vi "Send Email.vi"(8 "error in":errorcluster, 9 "Email Configuration":T2={"Subject"="Checking the Toolkit", "Body"="Please reply!", "Recipients Email Addresses"="", "CC - Optional"=[""]}, 10 "Sender's Configuration":T1={"Outgoing Mail Server (SMTP)"="smtp.gmail.com", "Port"=587, "Sender's Email"="", "Email Password"="", "Sender's Name"=""}, 11 "Attachment(optional)":path) -> (0 "error out":errorcluster)   [LabVIEW 2016]
doc: "Send Email VI sends email to specified accounts(depending on the server and port mentioned) with an optional attachment. Note that the default settings are for Gmail."
uses:
  controls/Email Configuration.ctl
  controls/Receipants Email Address.ctl
  controls/Sender's Configuration.ctl
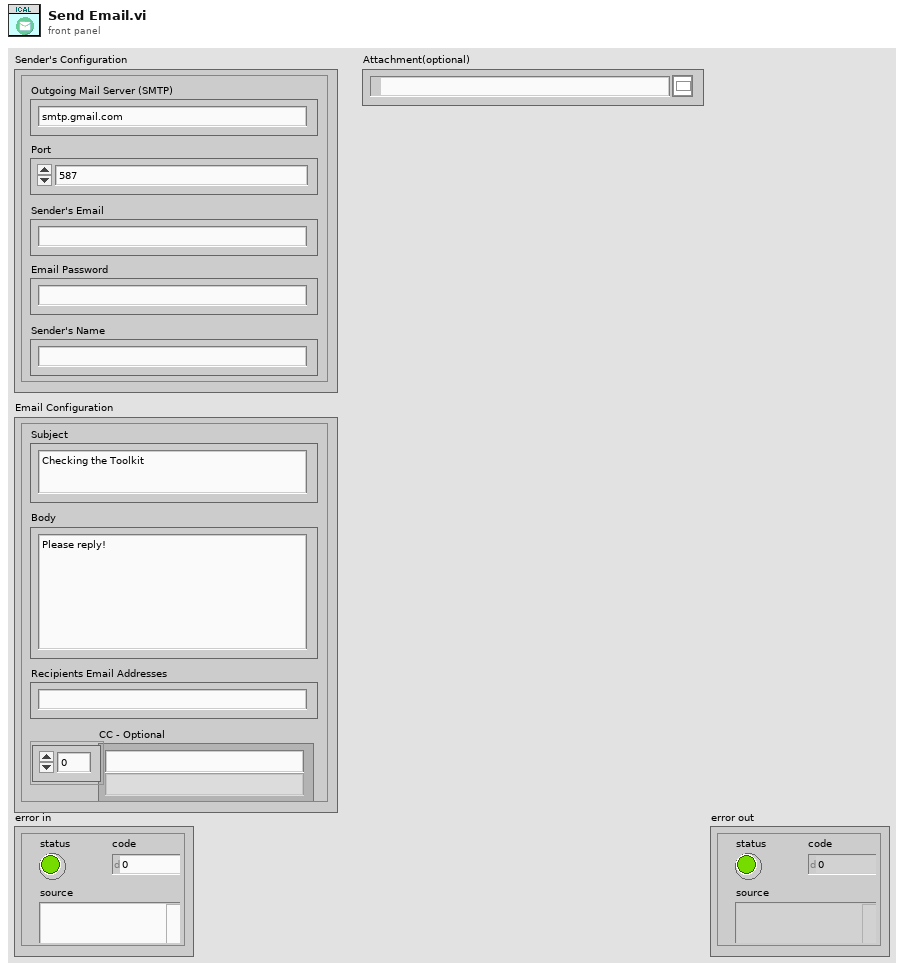
[diagram p1: front panel]
types:
  T1 = typedef "Sender's Configuration.ctl" = cluster{"Outgoing Mail Server (SMTP)":string, "Port":i32, "Sender's Email":string, "Email Password":string, "Sender's Name":string}
  T2 = typedef "Email Configuration.ctl" = cluster{"Subject":string, "Body":string, "Recipients Email Addresses":T3, "CC - Optional":string[]}
  T3 = typedef "Receipants Email Address.ctl" = string
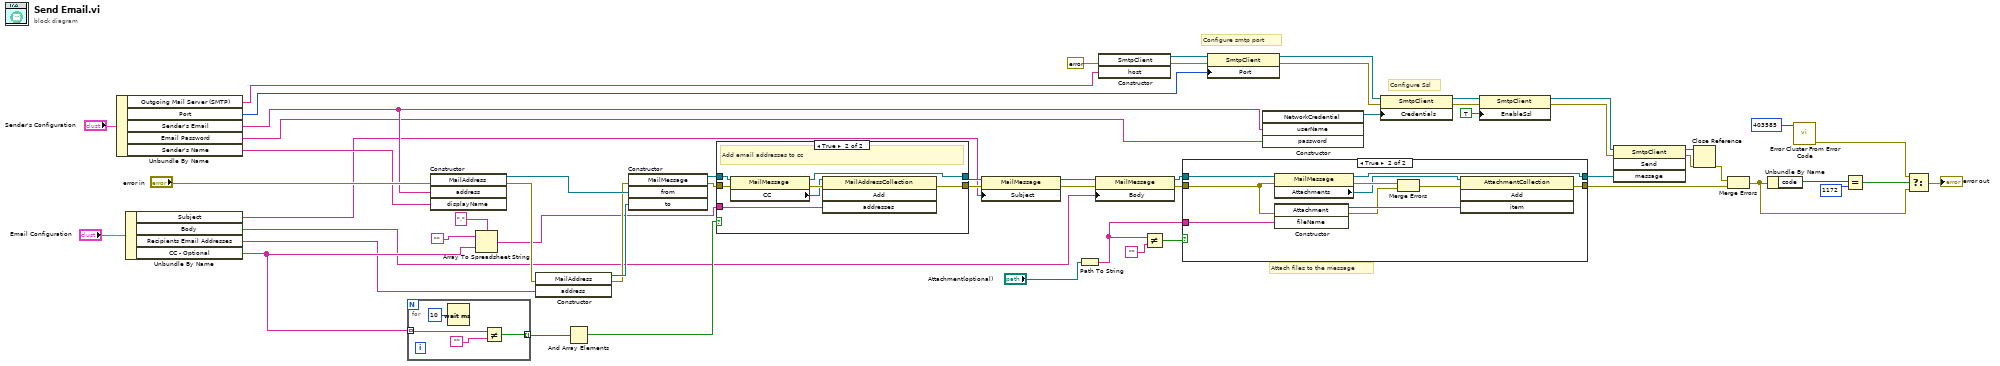
[diagram p0: block diagram]
diagram:
  # "Attach files to the message"
  # "Configure Ssl"
  # "Configure smtp port"
  n1 = Unbundle By Name("Sender's Configuration") -> ("Outgoing Mail Server (SMTP)"=w9:string, "Port"=w8:i32, "Sender's Email"=w7:string, "Email Password"=w5:string, "Sender's Name"=w6:string)
  n2 = Unbundle By Name("Email Configuration") -> ("Subject"=w1:string, "Body"=w2:string, "Recipients Email Addresses"=w3:T3, "CC - Optional"=w4:string[])
  n3 = for {
    tunnel: w4 -> [w58] mode=indexing
    tunnel: [w59] -> w18 mode=indexing
    n4 = Wait (ms)(milliseconds to wait=u32 10) -> ()  [unwired: 1 out]
    n5 = Not Equal?(x=w58, y="") -> (x != y?=w59:bool)
  }
  n6 = constructor class="MailAddress"(error in="error in", "address"=w7, "displayName"=w6) -> (reference out=w55:refnum<k24>, error out=w56:errorcluster)  [unwired: 2 in, 3 out]
  n7 = Array To Spreadsheet String(delimiter (Tab)=",", array=w4, 3:"" ("y")) -> (spreadsheet string=w19:string)
  n8 = constructor class="MailAddress"(error in=w56, "address"=w3) -> (reference out=w27:refnum<k24>, error out=w26:errorcluster)  [unwired: 2 in, 2 out]
  n9 = And Array Elements(Boolean array=w18) -> (logical AND=w17:bool)
  n10 = constructor class="MailMessage"(error in=w26, "from"=w55, "to"=w27) -> (reference out=w33:refnum<k24>, error out=w34:errorcluster)  [unwired: 2 in, 3 out]
  n11 = case shown="True" w17 {
    tunnel: w33 -> [w62 w67]
    tunnel: w34 -> [w61 w66]
    tunnel: [w62 w65] -> w32
    tunnel: [w61 w64] -> w31
    tunnel: w19 -> [_ w63]
    frame False {
    }
    frame True {
      # "Add email addresses to cc"
      n12 = property class="MailMessage"(reference=w67, error in=w66) -> (reference out=w65:refnum<k24>, error out=w69:errorcluster, "CC"=w68:refnum<k24>)
      n13 = invoke class="MailAddressCollection" method="Add"(reference=w68, error in=w69, "addresses"=w63) -> (error out=w64:errorcluster)  [unwired: 1 in, 3 out]
    }
  }
  n14 = property class="MailMessage"(reference=w32, error in=w31, "Subject"=w1) -> (reference out=w48:refnum<k24>, error out=w47:errorcluster)
  n15 = Path To String(path="Attachment(optional)") -> (string=w52:string)
  n16 = property class="MailMessage"(reference=w48, error in=w47, "Body"=w2) -> (reference out=w49:refnum<k24>, error out=w53:errorcluster)
  n17 = constructor class="SmtpClient"(error in=errorcluster {"status"=FALSE, "code"=0, "source"=""} ("error in (no error)"), "host"=w9) -> (reference out=w39:refnum<k24>, error out=w42:errorcluster)  [unwired: 2 in, 2 out]
  n18 = Not Equal?(x=w52, y="") -> (x != y?=w51:bool)
  n19 = case shown="True" w51 {
    tunnel: w49 -> [w71 w78]
    tunnel: [w71 w77] -> w35
    tunnel: w52 -> [_ w76]
    tunnel: w53 -> [w70 w75]
    tunnel: [w70 w72] -> w29
    frame False {
    }
    frame True {
      n20 = property class="MailMessage"(reference=w78, error in=w75) -> (reference out=w77:refnum<k24>, error out=w81:errorcluster, "Attachments"=w79:refnum<k24>)
      n21 = constructor class="Attachment"(error in=w75, "fileName"=w76) -> (reference out=w80:refnum<k24>, error out=w73:errorcluster)  [unwired: 2 in, 2 out]
      n22 = Merge Errors(w81, w73) -> (w74:errorcluster)
      n23 = invoke class="AttachmentCollection" method="Add"(reference=w79, error in=w74, "item"=w80) -> (error out=w72:errorcluster)  [unwired: 1 in, 3 out]
    }
  }
  n24 = property class="SmtpClient"(reference=w39, error in=w42, "Port"=w8) -> (reference out=w40:refnum<k24>, error out=w43:errorcluster)
  n25 = constructor class="NetworkCredential"("userName"=w7, "password"=w5) -> (reference out=w38:refnum<k24>)  [unwired: 3 in, 4 out]
  n26 = property class="SmtpClient"(reference=w40, error in=w43, "Credentials"=w38) -> (reference out=w41:refnum<k24>, error out=w44:errorcluster)
  n27 = property class="SmtpClient"(reference=w41, error in=w44, "EnableSsl"=TRUE) -> (reference out=w46:refnum<k24>, error out=w45:errorcluster)
  n28 = invoke class="SmtpClient" method="Send"(reference=w46, error in=w45, "message"=w35) -> (reference out=w37:refnum<k24>, error out=w36:errorcluster)  [unwired: 1 in, 2 out]
  n29 = Close Reference(reference=w37, error in (no error)=w36) -> (error out=w30:errorcluster)
  n30 = Merge Errors(w30, w29) -> (w13:errorcluster)
  n31 = Unbundle By Name(w13) -> ("code"=w16:i32)
  n32 = call <vilib>:"Error Cluster From Error Code.vi"("error code (0)"=403585 ("code")) -> ("error out"=w12:errorcluster)  [unwired: 8 in]
  n33 = Equal?(x=w16, y=1172) -> (x = y?=w14:bool)
  n34 = Select(t=w12, s=w14, f=w13) -> (s? t:f=→"error out":errorcluster)
